vi "XML.StringToControlVariant.vi"(8 "error in (no error)":errorcluster, 10 "node text":string, 11 "Control in":refnum<vi>) -> (0 "error out":errorcluster, 2 "Variant":variant, 3 "Control out":refnum<vi>)   [LabVIEW 2019, in "Tools.lvlib"]
uses:
  Tools.lvlib
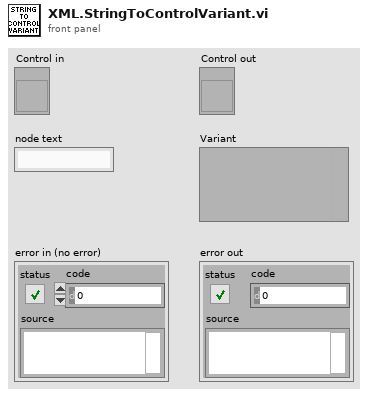
[diagram p1: front panel]
types:
  T1 = typedef "LVStringsAndValuesArrayTypeDef.ctl" = cluster{"String":string, "Value":ext}[]
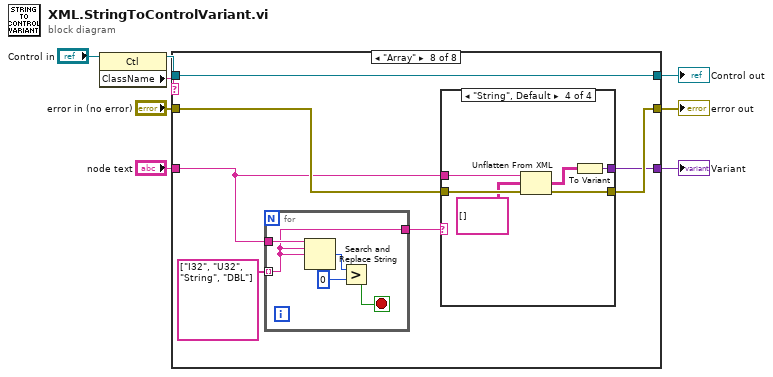
[diagram p0: block diagram]
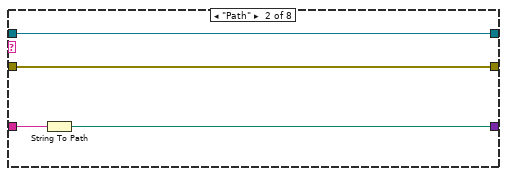
[diagram p3: hidden frame]
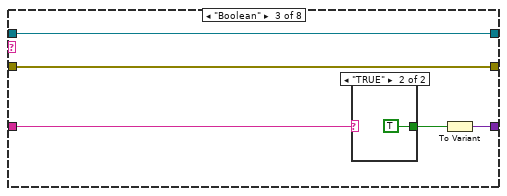
[diagram p4: hidden frame]
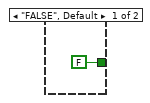
[diagram p5: hidden frame]
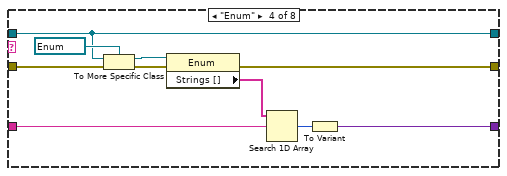
[diagram p6: hidden frame]
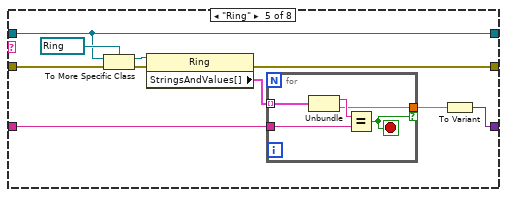
[diagram p7: hidden frame]
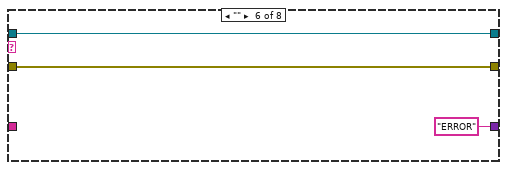
[diagram p8: hidden frame]
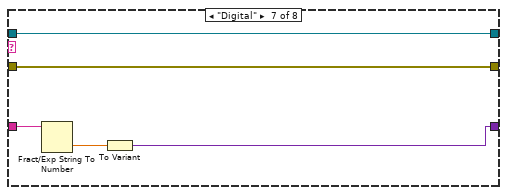
[diagram p9: hidden frame]
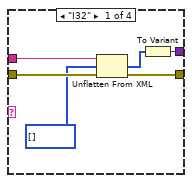
[diagram p10: hidden frame]
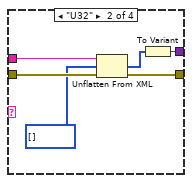
[diagram p11: hidden frame]
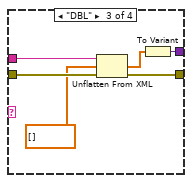
[diagram p12: hidden frame]
diagram:
  n1 = property class="Ctl"(reference="Control in") -> (reference out=w1:refnum<vi>, "ClassName"=w3:string)  [unwired: 1 in, 1 out]
  n2 = case shown="\"Array\"" w3 {
    tunnel: "node text" -> [w11 w15 w20 w29 w36 _ w55 w58]
    tunnel: [w11 w14 w18 w26 w37 "ERROR" w53 w57] -> w5
    tunnel: w1 -> [w10 w13 w17 w25 w35 w49 w52 w56]
    tunnel: [w10 w13 w17 w25 w35 w49 w52 w56] -> w6
    tunnel: "error in (no error)" -> [w9 w12 w16 w24 w34 w48 w51 w59]
    tunnel: [w9 w12 w16 w23 w33 w48 w51 w60] -> w8
    frame "ComboBox", "DAQmxName", "IVILogicalName", "String", "VISAResourceName", Default {
    }
    frame "Path" {
      n3 = String To Path(string=w15) -> (path=w14:path)
    }
    frame "Boolean" {
      n4 = case shown="\"TRUE\"" w20 {
        tunnel: [FALSE TRUE] -> w19
        frame "FALSE", Default {
        }
        frame "TRUE" {
        }
      }
      n5 = To Variant(anything=w19) -> (Variant=w18:variant)
    }
    frame "Enum" {
      n6 = To More Specific Class(target class=refnum<vi> refnum ("TESTITEM"), reference=w25, error in=w24) -> (specific class reference=w31:refnum<vi>, error out=w32:errorcluster)
      n7 = property class="Enum"(reference=w31, error in=w32) -> (error out=w23:errorcluster, "Strings []"=w28:string[])  [unwired: 1 out]
      n8 = Search 1D Array(1D array=w28, element=w29) -> (index of element=w27:i32)  [unwired: 1 in]
      n9 = To Variant(anything=w27) -> (Variant=w26:variant)
    }
    frame "Ring" {
      n10 = To More Specific Class(target class=refnum<vi> refnum ("TESTITEM"), reference=w35, error in=w34) -> (specific class reference=w41:refnum<vi>, error out=w42:errorcluster)
      n11 = property class="Ring"(reference=w41, error in=w42) -> (error out=w33:errorcluster, "StringsAndValues[]"=w39:T1)  [unwired: 1 out]
      n12 = for {
        tunnel: w39 -> [w47] mode=indexing
        tunnel: [w44] -> w38 if=w43
        tunnel: w36 -> [w45]
        stop <- w43 stop-if-true
        n13 = Unbundle(w47) -> ("String"=w46:string, "Value"=w44:ext)
        n14 = Equal?(x=w46, y=w45) -> (x = y?=w43:bool)
      }
      n15 = To Variant(anything=w38) -> (Variant=w37:variant)
    }
    frame "" {
    }
    frame "Digital" {
      n16 = Fract/Exp String To Number(string=w55) -> (number=w54:dbl)  [unwired: 3 in, 1 out]
      n17 = To Variant(anything=w54) -> (Variant=w53:variant)
    }
    frame "Array" {
      n18 = for {
        tunnel: w58 -> [w91]
        tunnel: string[] ["I32", "U32", "String", "DBL"] -> [w90] mode=indexing
        tunnel: [w90] -> w61
        stop <- w87 stop-if-true
        n19 = Search and Replace String(input string=w91, search string=w90, replace string=w90) -> (number of replacements=w89:i32)  [unwired: 5 in, 3 out]
        n20 = Greater?(x=w89, y=0) -> (0:w87:bool)
      }
      n21 = case shown="\"String\", Default" w61 {
        tunnel: [w67 w73 w79 w85] -> w60
        tunnel: w59 -> [w66 w72 w78 w84]
        tunnel: w58 -> [w65 w71 w77 w83]
        tunnel: [w64 w70 w76 w82] -> w57
        frame "I32" {
          n22 = Unflatten From XML(xml string=w65, type=i32[] [], error in (no error)=w66) -> (value=w68:i32[], error out=w67:errorcluster)
          n23 = To Variant(anything=w68) -> (Variant=w64:variant)
        }
        frame "U32" {
          n24 = Unflatten From XML(xml string=w71, type=u32[] [], error in (no error)=w72) -> (value=w74:u32[], error out=w73:errorcluster)
          n25 = To Variant(anything=w74) -> (Variant=w70:variant)
        }
        frame "DBL" {
          n26 = Unflatten From XML(xml string=w77, type=dbl[] [], error in (no error)=w78) -> (value=w80:dbl[], error out=w79:errorcluster)
          n27 = To Variant(anything=w80) -> (Variant=w76:variant)
        }
        frame "String", Default {
          n28 = Unflatten From XML(xml string=w83, type=string[][] [], error in (no error)=w84) -> (value=w86:string[][], error out=w85:errorcluster)
          n29 = To Variant(anything=w86) -> (Variant=w82:variant)
        }
      }
    }
  }
  "error out" <- w8
  "Control out" <- w6
  "Variant" <- w5
